vi "First Identity.vi"(5 "Username":string, 6 "Password":string, 7 "Address":string, 8 "Error In":errorcluster) -> (0 "Error Out":errorcluster)   [LabVIEW 2018, in "Tests.lvlib" / "Agent.lvlib"]
uses:
  Agent.lvlib
  <vilib>/addons/_JKI Toolkits/Caraya/classes/Test/Test.lvclass
  <vilib>/addons/_JKI Toolkits/Caraya/classes/Assert/Assert.lvclass
  src/Toolkit/Agent/Agent.lvclass
  src/Toolkit/Agent Identity/Agent Identity.lvclass
  src/Toolkit/Agent Identity/Support/Create from Agent.vi
  src/Toolkit/Agent Identity/Support/Destroy to Agent.vi
  src/Toolkit/Agent/API/Typedefs/Results.ctl
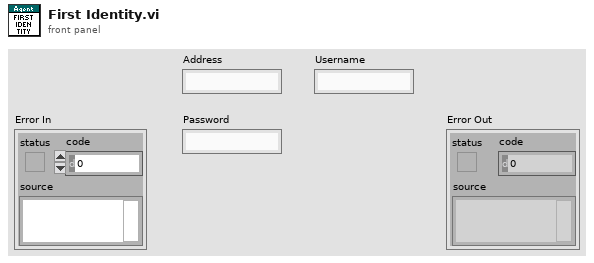
[diagram p1: front panel]
types:
  T1 = typedef "Toolkit.lvlib/Agent.lvclass/Results.ctl" = enum32{"Success", "End of Identities"}
  T2 = typedef "Toolkit.lvlib/Agent.lvclass/Results.ctl" = i32
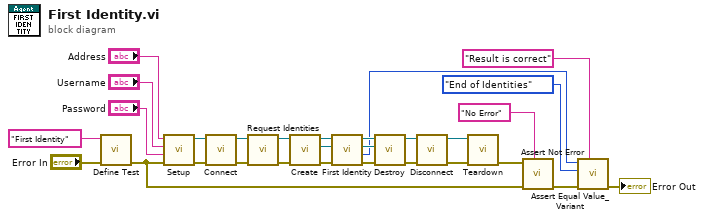
[diagram p0: block diagram]
diagram:
  n1 = call <vilib>:"Define Test.vi"("error in (no error)"="Error In", "Label (VI Title)"="First Identity") -> ("error out"=w23:errorcluster)  [unwired: 9 in]
  n2 = call "Setup.vi"("Error In"=w23, "Password"="Password", "Username"="Username", "Address"="Address") -> ("Error Out"=w21:errorcluster, "Agent"=w22:refnum<class "Agent.lvclass">)  [unwired: 6 in]
  n3 = call "Connect.vi"("Error In"=w21, "Agent In"=w22) -> ("Error Out"=w19:errorcluster, "Agent Out"=w20:refnum<class "Agent.lvclass">)  [unwired: 8 in]
  n4 = call "Request Identities.vi"("Error In"=w19, "Agent In"=w20) -> ("Error Out"=w17:errorcluster, "Agent Out"=w18:refnum<class "Agent.lvclass">)  [unwired: 8 in]
  n5 = call-poly "Create.vi"("Error In"=w17, "Agent In"=w18) -> ("Error Out"=w15:errorcluster, "Identity"=w14:refnum<class "Agent Identity.lvclass">, "Agent Out"=w16:refnum<class "Agent.lvclass">)  [unwired: 7 in]
  n6 = call "First Identity.vi"("Error In"=w15, "Identity In"=w14, "Agent In"=w16) -> ("Error Out"=w12:errorcluster, "Result"=w9:T2, "Identity Out"=w11:refnum<class "Agent Identity.lvclass">, "Agent Out"=w13:refnum<class "Agent.lvclass">)  [unwired: 5 in]
  n7 = call-poly "Destroy.vi"("Error In"=w12, "Identity"=w11, "Agent In"=w13) -> ("Error Out"=w6:errorcluster, "Agent Out"=w7:refnum<class "Agent.lvclass">)  [unwired: 7 in]
  n8 = call "Disconnect.vi"("Error In"=w6, "Agent In"=w7) -> ("Error Out"=w5:errorcluster, "Agent Out"=w4:refnum<class "Agent.lvclass">)  [unwired: 8 in]
  n9 = call "Teardown.vi"("Error In"=w5, "Agent"=w4) -> ("Error Out"=w10:errorcluster)  [unwired: 9 in]
  n10 = call <vilib>:"Assert Not Error.vi"("Label"="No Error", "error in (no error)"=w23, "Not Error?"=w10) -> ("error out"=w26:errorcluster)  [unwired: 8 in]
  n11 = call <vilib>:"Assert Equal Value_Variant.vi"("Label"="Result is correct", "error in (no error)"=w26, "Y"=Results."End of Identities" ("Result"), "X"=w9) -> ("error out"=→"Error Out":errorcluster)  [unwired: 7 in]
